vi "BusB_Stop Acquisition.vi"(8 "error in (no error)":errorcluster, 10 "HW Refnum":string, 11 "BusB Visa Resource":refnum<visa-resource-name>) -> (0 "error out":errorcluster)   [LabVIEW 2016, in "Impedance Data Acquisition and Decoding.lvlib"]
uses:
  Impedance Data Acquisition and Decoding.lvlib
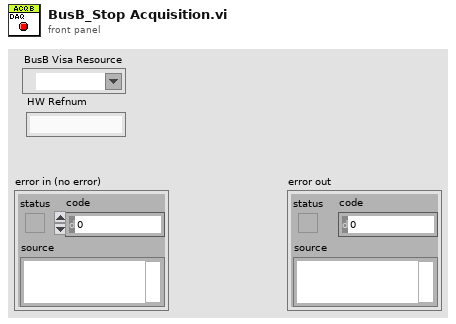
[diagram p1: front panel]
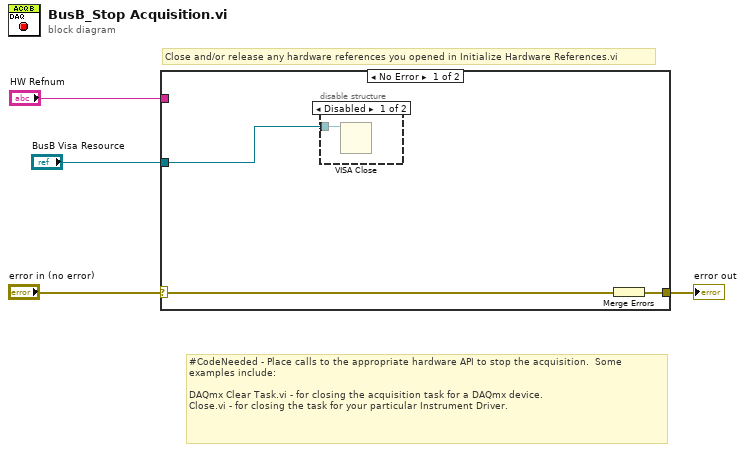
[diagram p0: block diagram]
diagram:
  # "#CodeNeeded - Place calls to the appropriate hardware API to stop the acquisition.  Some examples include:\n\nDAQmx Clear Task.vi - for closing the acquisition task for a DAQmx device.\nClose.vi - for closing the task for your particular Instrument Driver."
  # "Close and/or release any hardware references you opened in Initialize Hardware References.vi"
  n1 = case shown="No Error" "error in (no error)" {
    selector: "error in (no error)" -> [w5 w9]
    tunnel: [w7 w9] -> w3
    tunnel: "HW Refnum" -> [_ _]
    tunnel: "BusB Visa Resource" -> [w6 _]
    frame No Error {
      n2 = disable-structure shown="Disabled" {
        disable-tunnel: w6 -> [w8 _]
        frame Disabled {
          n3 = VISA Close(VISA resource name=w8) -> ()  [unwired: 1 in, 1 out]
        }
        frame Enabled {
        }
      }
      n4 = Merge Errors(w5) -> (w7:errorcluster)
    }
    frame Error {
    }
  }
  "error out" <- w3
